vi "Open Door.vi"(8 "error in (no error)":errorcluster, 11 "Doors Closing in":refnum<class "Doors Closing.lvclass">) -> (0 "error out":errorcluster, 3 "Doors Closing out":refnum<class "Doors Closing.lvclass">)   [LabVIEW 2020, in "Door Controller.lvlib" / "Doors Closing.lvclass"]
uses:
  Doors Closing.lvclass
  C:/Users/Thomas.McQuillan/Desktop/Elevator Door Control/Door Controller/Door Controller/Door Controller.lvclass
  Door Controller/Door Controller.lvclass/Door Controller.ctl
  <vilib>/ActorFramework/Message Enqueuer/Message Enqueuer.lvclass/Message Enqueuer.ctl
  <vilib>/ActorFramework/Message Enqueuer/Enqueue.vi
  Door Hardware/Door Hardware Messages/Open Doors Msg/Open Doors Msg.lvclass
  C:/Program Files/National Instruments/LabVIEW 2020/vi.lib/ActorFramework/Message/Message.lvclass
  <vilib>/ActorFramework/Message Priority Queue/Priority Enqueue.vi
  Door Controller/Door Controller.lvclass
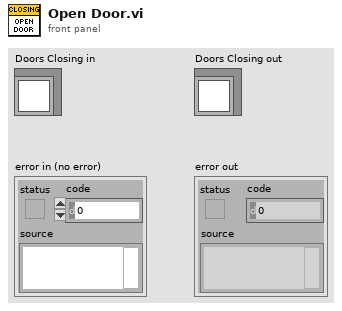
[diagram p1: front panel]
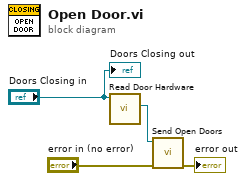
[diagram p0: block diagram]
diagram:
  n1 = call "Read Door Hardware.vi"("Door Controller in"="Doors Closing in") -> ("Door Hardware"=w4:refnum<class "Message Enqueuer.lvclass">)  [unwired: 10 in]
  n2 = call "Send Open Doors.vi"("error in (no error)"="error in (no error)", "Message Enqueuer"=w4) -> ("error out"=→"error out":errorcluster)  [unwired: 8 in, 1 out]
  "Doors Closing out" <- "Doors Closing in"
